vi "Get Consumer Values.vi"(8 "error in":errorcluster, 11 "Chiller Cluster.lvclass in":refnum<class "Chiller Cluster.lvclass">) -> (0 "error out":errorcluster, 1 "Consumer Ch":T1[](array[typedef]), 2 "Consumer Control":T2, 3 "Chiller Cluster.lvclass out":refnum<class "Chiller Cluster.lvclass">)   [LabVIEW 2023, in "Chiller Cluster.lvclass"]
uses:
  Chiller Cluster.lvclass
  Consumer Control.ctl
  Consumer Ch.ctl
  Chiller Cluster.lvclass/Chiller Cluster.ctl
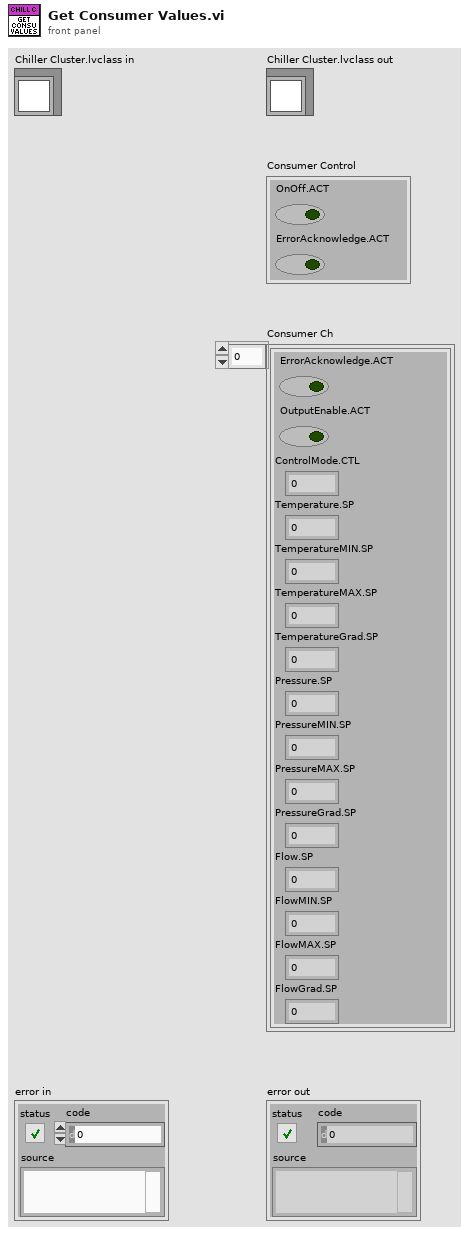
[diagram p1: front panel]
types:
  T1 = typedef "Chiller Cluster.lvclass/Consumer Ch.ctl" = cluster{"ErrorAcknowledge.ACT":bool, "OutputEnable.ACT":bool, "ControlMode.CTL":u16, "Temperature.SP":dbl, "TemperatureMIN.SP":dbl, "TemperatureMAX.SP":dbl, "TemperatureGrad.SP":dbl, "Pressure.SP":dbl, "PressureMIN.SP":dbl, "PressureMAX.SP":dbl, "PressureGrad.SP":dbl, "Flow.SP":dbl, "FlowMIN.SP":dbl, "FlowMAX.SP":dbl, "FlowGrad.SP":dbl}
  T2 = typedef "Chiller Cluster.lvclass/Consumer Control.ctl" = cluster{"OnOff.ACT":bool, "ErrorAcknowledge.ACT":bool}
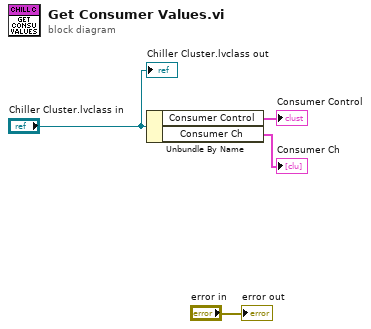
[diagram p0: block diagram]
diagram:
  n1 = Unbundle By Name("Chiller Cluster.lvclass in") -> ("Consumer Control"=→"Consumer Control":T2, "Consumer Ch"=→"Consumer Ch":T1[])
  "Chiller Cluster.lvclass out" <- "Chiller Cluster.lvclass in"
  "error out" <- "error in"
